vi "DM_Voltage.vi"(4 "error in":errorcluster caption="错误输入", 6 "add":u8=3 format="%.0x", 7 "MyIndex":u8) -> (0 "错误输出":errorcluster, 2 "OK?":bool, 3 "Value":dbl)   [LabVIEW 2015]
uses:
  <vilib>/Instr/_visa.llb/VISA Configure Serial Port (Instr).vi
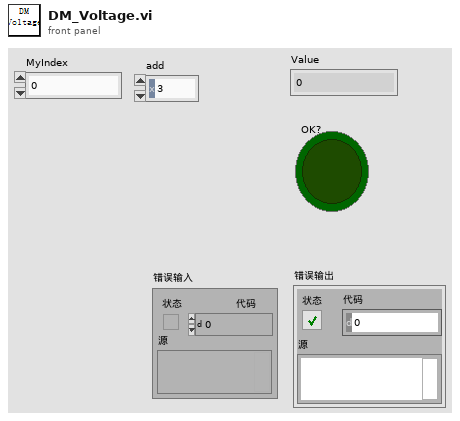
[diagram p1: front panel]
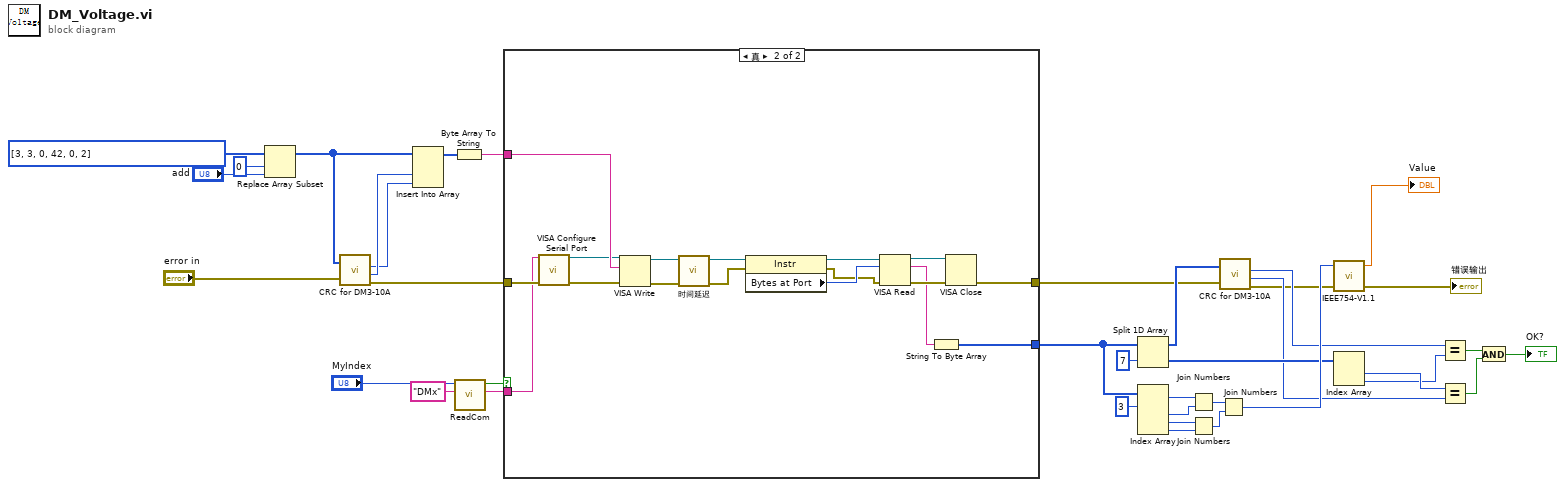
[diagram p0: block diagram]
diagram:
  n1 = Replace Array Subset(array=u8[] [3, 3, 0, 42, 0, 2] ("输入指令"), new element="add", index=0) -> (w6:u8[])
  n2 = call "CRC for DM3-10A.vi"("CMD"=w6, "error in (no error)"="error in") -> ("CRCHi"=w34:u8, "CRCLo"=w35:u8, "error out"=w12:errorcluster)  [unwired: 1 out]
  n3 = Insert Into Array(array=w6, new element #1=w35, new element #2=w34) -> (w36:u8[])  [unwired: 1 in]
  n4 = Byte Array To String(unsigned byte array=w36) -> (string=w37:string)
  n5 = call "ReadCom.vi"("仪器名称"="DMx", "MyIndex"="MyIndex") -> ("COM"=w2:string, "OK?"=w1:bool)  [unwired: 7 in, 1 out]
  n6 = case shown="真" w1 {
    tunnel: w37 -> [_ w50]
    tunnel: [_ w44] -> w23
    tunnel: w12 -> [w38 w43]
    tunnel: [w38 w42] -> w10
    tunnel: w2 -> [_ w41]
    frame False {
    }
    frame True {
      n7 = call-poly "VISA Configure Serial Port"("VISA resource name"=w41, "error in (no error)"=w43) -> ("VISA resource name out"=w49:refnum<visa-resource-name>, "error out"=w54:errorcluster)  [unwired: 12 in]
      n8 = VISA Write(VISA resource name=w49, write buffer=w50, error in (no error)=w54) -> (VISA resource name out=w48:refnum<visa-resource-name>, error out=w40:errorcluster)  [unwired: 1 out]
      n9 = call "时间延迟"("error in (no error)"=w40) -> ("error out"=w39:errorcluster)  [unwired: 10 in]
      n10 = property class="Instr"(reference=w48, error in=w39) -> (reference out=w45:refnum<visa-resource-name>, error out=w46:errorcluster, "Bytes at Port"=w47:u32)
      n11 = VISA Read(VISA resource name=w45, byte count=w47, error in (no error)=w46) -> (VISA resource name out=w52:refnum<visa-resource-name>, read buffer=w51:string, error out=w53:errorcluster)  [unwired: 1 out]
      n12 = String To Byte Array(string=w51) -> (unsigned byte array=w44:u8[])
      n13 = VISA Close(VISA resource name=w52, error in (no error)=w53) -> (error out=w42:errorcluster)
    }
  }
  n14 = Split 1D Array(array=w23, index=7 ("索引")) -> (first subarray=w21:u8[], second subarray=w20:u8[])
  n15 = Index Array(array=w23, index #1=3 ("索引")) -> (element #1=w31:u8, element #2=w32:u8, element #3=w30:u8, element #4=w29:u8)  [unwired: 3 in]
  n16 = Join Numbers(hi=w31, lo=w32) -> ((hi.lo)=w28:u16)
  n17 = Join Numbers(hi=w30, lo=w29) -> ((hi.lo)=w27:u16)
  n18 = Join Numbers(hi=w28, lo=w27) -> ((hi.lo)=w26:u32)
  n19 = call "CRC for DM3-10A.vi"("CMD"=w21, "error in (no error)"=w10) -> ("CRCHi"=w19:u8, "CRCLo"=w18:u8, "error out"=w9:errorcluster)  [unwired: 1 out]
  n20 = call "IEEE754-V1.1.vi"("error in (no error)"=w9, "数字"=w26) -> ("error out"=→"错误输出":errorcluster, "输出浮点型"=→"Value":dbl)  [unwired: 2 in]
  n21 = Index Array(array=w20) -> (element #1=w14:u8, element #2=w13:u8)  [unwired: 2 in]
  n22 = Equal?(x=w19, y=w13) -> (x = y?=w17:bool)
  n23 = Equal?(x=w14, y=w18) -> (x = y?=w16:bool)
  n24 = And(x=w17, y=w16) -> (x .and. y?=→"OK?":bool)
